vi "MovePuzzlePeices.vi"(4 "Upper White Row Position":i32, 5 "Solved Puzzle":picture[][](array[picture]), 7 "Current Puzzle State":picture[][](array[picture]), 8 "Current Selected Peice Column":i32, 9 "Current Selected Peice Row":i32, 10 "Lower White Coordinate":i32, 11 "Allow Peice Movement":bool) -> (2 "Puzzle Finished":bool, 3 "Updated Image Array":picture[][](array[picture]))   [LabVIEW 2014]
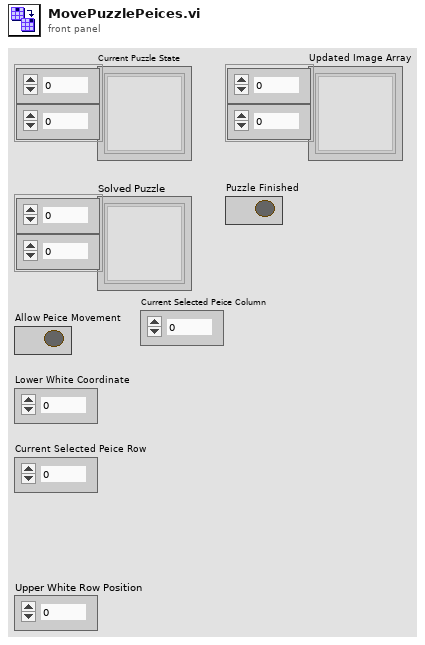
[diagram p1: front panel]
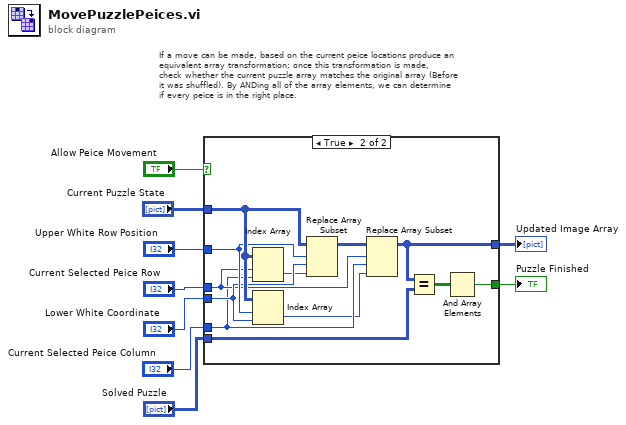
[diagram p0: block diagram]
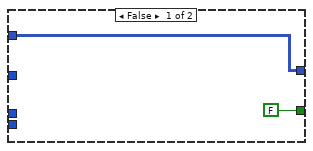
[diagram p2: hidden frame]
diagram:
  # "If a move can be made, based on the current peice locations produce an\nequivalent array transformation; once this transformation is made,\ncheck whether the current puzzle array matches the original array (Before\nit was shuffled). By ANDing all of the array elements, we can determine\nif every peice is in the right place."
  n1 = case shown="True" "Allow Peice Movement" {
    tunnel: "Current Puzzle State" -> [w11 w23]
    tunnel: "Upper White Row Position" -> [_ w22]
    tunnel: "Lower White Coordinate" -> [_ w21]
    tunnel: "Current Selected Peice Row" -> [_ w18]
    tunnel: "Current Selected Peice Column" -> [_ w17]
    tunnel: [w11 w12] -> w6
    tunnel: "Solved Puzzle" -> [_ w13]
    tunnel: [FALSE w14] -> w9
    frame False {
    }
    frame True {
      n2 = Index Array(array=w23, index (row)=w18, index (col)=w17) -> (element=w20:picture)
      n3 = Index Array(array=w23, index (row)=w22, index (col)=w21) -> (element=w16:picture)
      n4 = Replace Array Subset(array=w23, new element=w20, index (row)=w22, index (col)=w21) -> (w19:picture[][])
      n5 = Replace Array Subset(array=w19, new element=w16, index (row)=w18, index (col)=w17) -> (w12:picture[][])
      n6 = Equal?(x=w12, y=w13) -> (x = y?=w15:bool[][])
      n7 = And Array Elements(Boolean array=w15) -> (logical AND=w14:bool)
    }
  }
  "Puzzle Finished" <- w9
  "Updated Image Array" <- w6
